vi "Click Cycle_Next Row State.vi"(8 "Error In":errorcluster, 11 "Current Row State":T1) -> (0 "Error Out":errorcluster, 3 "Next Row State":T1)   [LabVIEW 2023]
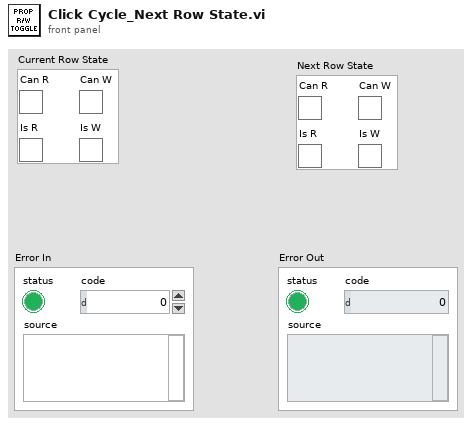
[diagram p1: front panel]
types:
  T1 = cluster{"Can R":bool, "Can W":bool, "Is R":bool, "Is W":bool}
  T2 = cluster{"Can R":bool, "Can W":bool, "Is R":bool, "Is W":bool}[]
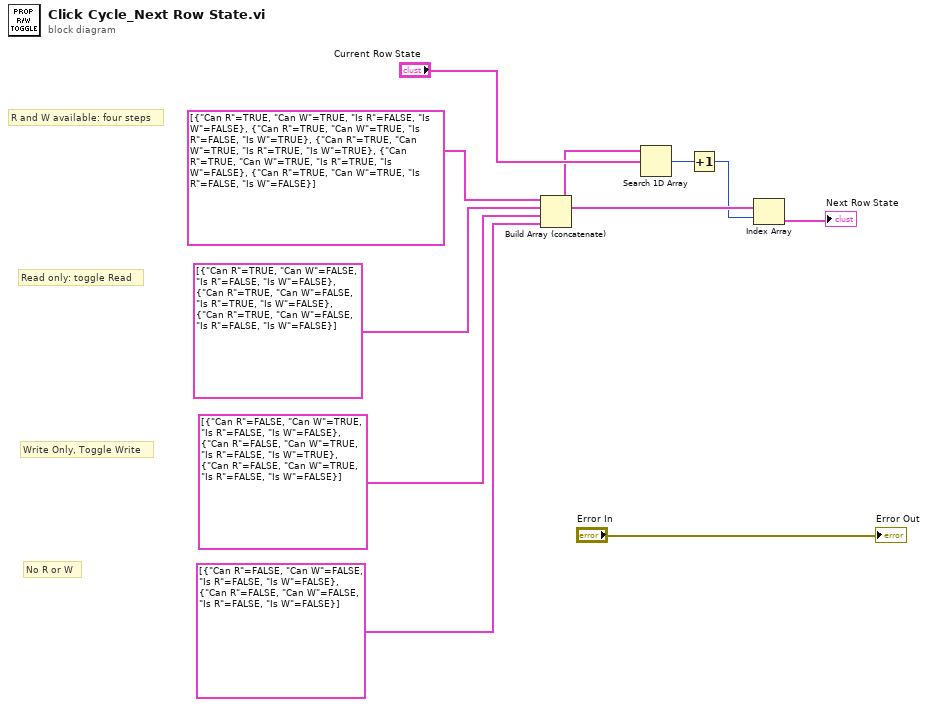
[diagram p0: block diagram]
diagram:
  # "No R or W"
  # "Write Only, Toggle Write"
  # "Read only: toggle Read"
  # "R and W available: four steps"
  n1 = Build Array (concatenate)(T2 [{"Can R"=TRUE, "Can W"=TRUE, "Is R"=FALSE, "Is W"=FALSE}, {"Can R"=TRUE, "Can W"=TRUE, "Is R"=FALSE, "Is W"=TRUE}, {"Can R"=TRUE, "Can W"=TRUE, "Is R"=TRUE, "Is W"=TRUE}, {"Can R"=TRUE, "Can W"=TRUE, "Is R"=TRUE, "Is W"=FALSE}, {"Can R"=TRUE, "Can W"=TRUE, "Is R"=FALSE, "Is W"=FALSE}], T2 [{"Can R"=TRUE, "Can W"=FALSE, "Is R"=FALSE, "Is W"=FALSE}, {"Can R"=TRUE, "Can W"=FALSE, "Is R"=TRUE, "Is W"=FALSE}, {"Can R"=TRUE, "Can W"=FALSE, "Is R"=FALSE, "Is W"=FALSE}], T2 [{"Can R"=FALSE, "Can W"=TRUE, "Is R"=FALSE, "Is W"=FALSE}, {"Can R"=FALSE, "Can W"=TRUE, "Is R"=FALSE, "Is W"=TRUE}, {"Can R"=FALSE, "Can W"=TRUE, "Is R"=FALSE, "Is W"=FALSE}], T2 [{"Can R"=FALSE, "Can W"=FALSE, "Is R"=FALSE, "Is W"=FALSE}, {"Can R"=FALSE, "Can W"=FALSE, "Is R"=FALSE, "Is W"=FALSE}]) -> (w6:T2)
  n2 = Search 1D Array(1D array=w6, element="Current Row State") -> (index of element=w5:i32)  [unwired: 1 in]
  n3 = Increment(x=w5) -> (x+1=w3:i32)
  n4 = Index Array(array=w6, index=w3) -> (element=→"Next Row State":T1)
  "Error Out" <- "Error In"
